vi "Door_position.vi"() -> ()   [LabVIEW 2016]
panel:
  in  "index":i32=2
  in  "BACK":bool
  out "array w/ subset deleted":string[](array[string])
  out "element":string
  in  "Array":string[](array[string])
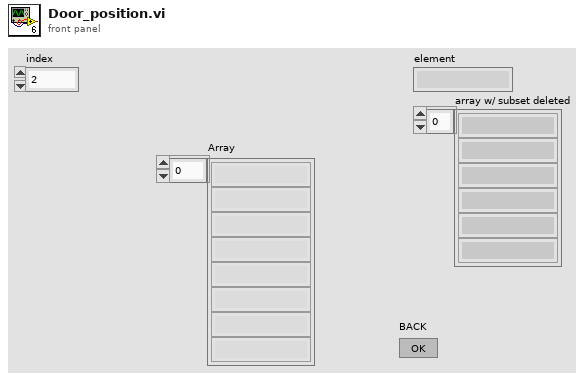
[diagram p1: front panel]
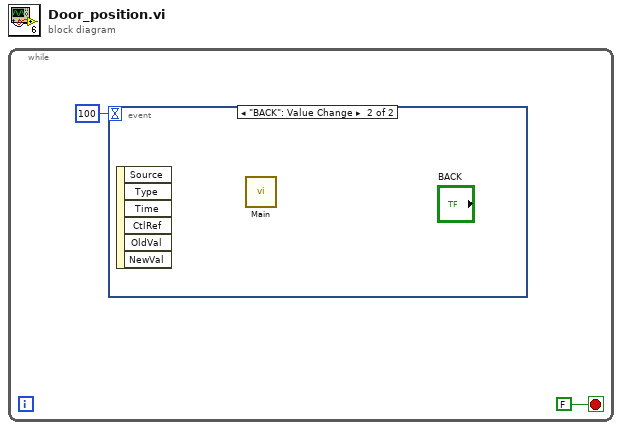
[diagram p0: block diagram]
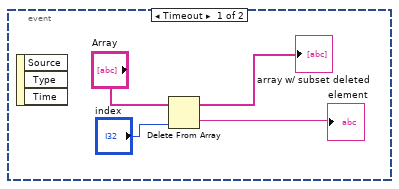
[diagram p2: hidden frame]
diagram:
  n1 = while {
    stop <- FALSE stop-if-true
    n2 = event shown="[1] \"BACK\": Value Change" {
      selector: _ -> [_ _]
      dyn-events: _ -> [_ _]
      timeout: 100 -> [_ _]
      event Timeout {
        n3 = event-data() -> ()  [unwired: 1 in, 3 out]
        n4 = Delete From Array(array="Array", index="index") -> (deleted portion=→"element":string, array with subset deleted=→"array w/ subset deleted":string[])  [unwired: 1 in]
      }
      event "BACK": Value Change {
        n5 = event-data() -> ()  [unwired: 1 in, 6 out]
        n6 = call "Main.vi"() -> ()  [unwired: 12 in]
      }
    }
  }
